vi "Agilent 546XX Series Acq Wfm Edge Triggered Oscilloscope Tapped.vi"(0 "VISA Resource Name":refnum<visa-resource-name> caption="VISA session", 1 "Vertical Coupling (DC)":i32(slide)=1, 2 "acquisition start time (0.0 sec)":dbl caption="Acquisition Start Time (0.0 sec)" format="%^.2e", 3 "probe attenuation (1.0)":dbl=1.0 caption="Probe Attenuation (1x)" format="%.2f", 5 "Channel Name (\"Channel 1\")":string(combo)="CHAN1", 7 "vertical range (40.0 V)":dbl=2.0 caption="Vertical Range (2.0 V)" format="%^.2e", 9 "time per record (1.00E-3 sec)":dbl=0.02 caption="Time Per Record (20.0E-3 sec)" format="%^.2e", 12 "trigger level (0.0 volts)":dbl caption="Trigger Level (0.0 volts)" format="%^.2e", 13 "minimum record length (2000)":i32=1000 caption="Min Record Length (1000 samples)", 14 "vertical offset (0.0 V)":dbl caption="Vertical Offset (0.0 V)" format="%^.2e") -> (6 "Waveform Graph":T1(graph))   [LabVIEW 2014]
doc: "DESCRIPTION:\nThis VI shows how to configure the ag546xx for a single-channel waveform acquisition. It uses edge triggering to trigger the acquisition. \n\nINSTRUCTIONS:\n1. Pass a valid instrument VISA session into this VI.\n2. Enter a vertical range and coupling for the specified channel.\n3. Enter the probe attenuation for the probe attached to the specified channel input.\n4. Enter the acquisition start time and desired time per record.\n5. Enter the trigger level for the edge trigger.\n6. Run the VI.\n7. The acquired waveform will be displayed in the graph.\n\nNOTES:\nNotice the order of the ag546xx component VIs in the block diagram. The first VI in this sequence accepts a valid instrument VISA session which provides a dup VISA session to the instrument driver. The instrument session is generated by the ag546xx Initialize.vi. The last VI in the sequence passes the VISA session out. \n\nThis VI sets the following controls on the block diagram:\n 60MHz Max Input Frequency.\n 1.0M Ohm Input Impedance.\n 200 ns Trigger Holdoff\n Edge trigger is DC coupled with a positive slope.\nTo change these values, modify the associated block diagram constants."
uses:
  <instrlib>/Agilent 546XX Series/Agilent 546XX Series.lvlib
panel:
  in  "Serial Configuration":cluster{"Baud Rate":u32, "Flow Control":u16}={"Baud Rate"=0, "Flow Control"=4} {"Flow Control" items=["None", "XON/XOFF", "RTS/CTS", "XON/XOFF & RTS/CTS", "DTR/DSR", "XON/XOFF & DTR/DSR"]; "Baud Rate" items=["9600", "19200", "38400", "57600"]}
  # "© 2003, National Instruments, Corporation.  All Rights Reserved."
  # "For instructions,\nselect Show Context Help\nfrom the Help menu."
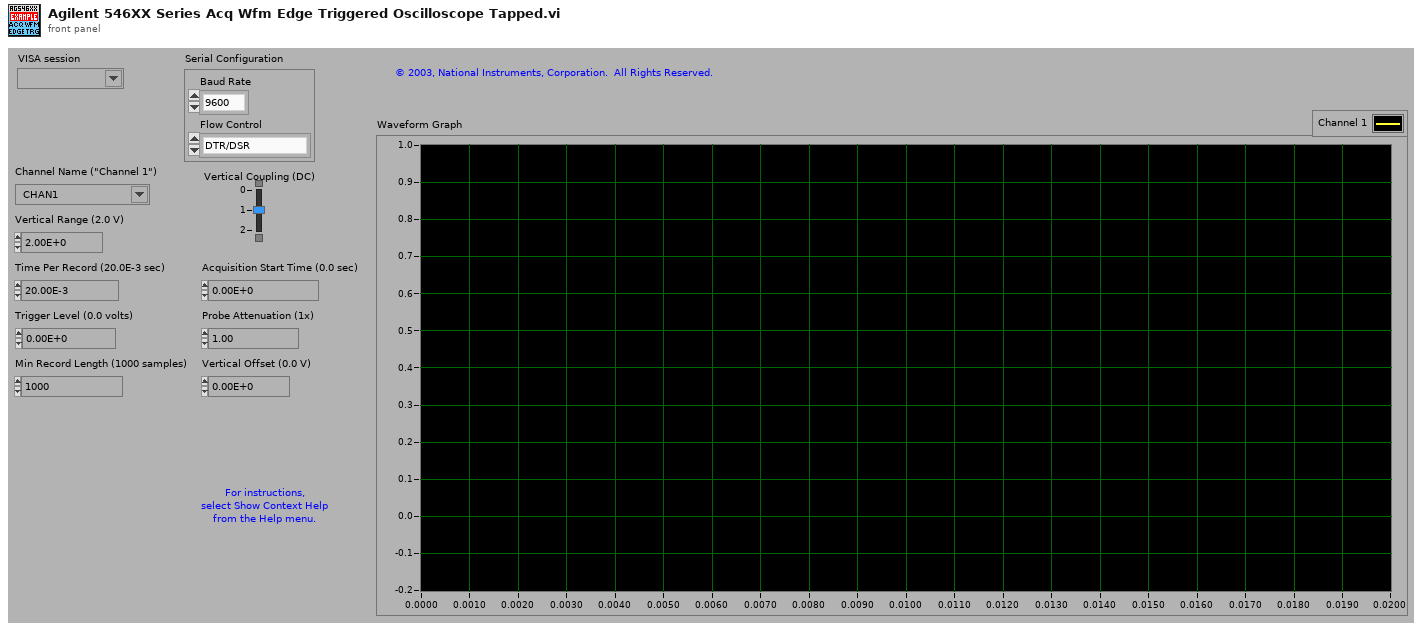
[diagram p1: front panel]
types:
  T1 = cluster{"Initial X":dbl, "X Increment":dbl, "Waveform Array":dbl[]}
  T2 = cluster{"initial x":dbl, "x increment":dbl, " waveform array  ":dbl[]}
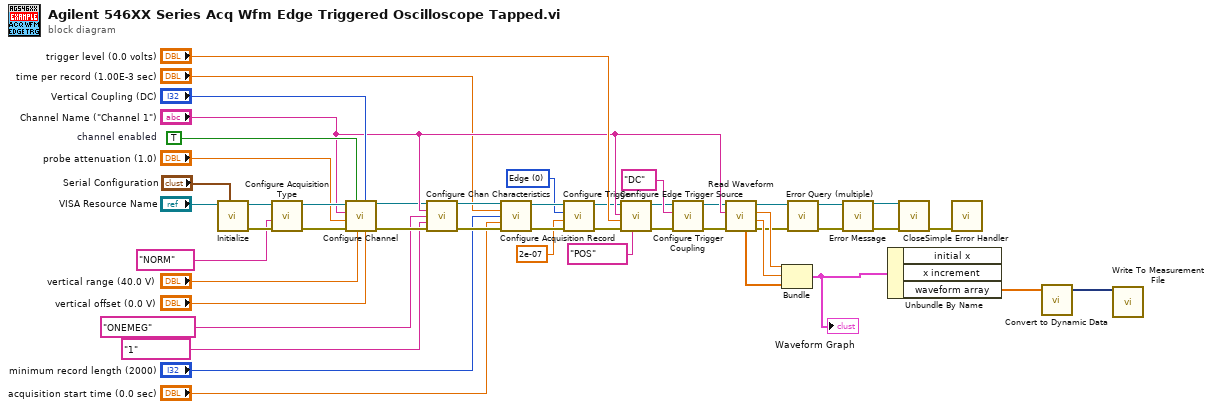
[diagram p0: block diagram]
diagram:
  w22 = 0 items=["Edge", "Glitch", "TV", "AC Line", "Pattern", "Duration", "IIC", "Sequence"] ("Trigger Type (Edge)")
  w39 = TRUE  # channel enabled
  n1 = call <instrlib>:"Initialize.vi"("Serial Configuration"="Serial Configuration", "VISA Resource Name"="VISA Resource Name") -> ("error out"=w48:errorcluster, "VISA Resource Name Out"=w12:refnum<visa-resource-name>)  [unwired: 8 in]
  n2 = call <instrlib>:"Configure Acquisition Type.vi"("error in (no error)"=w48, "Acquisition Type (Sample)"="NORM", "VISA Resource Name"=w12) -> ("error out"=w47:errorcluster, "VISA Resource Name Out"=w45:refnum<visa-resource-name>)  [unwired: 7 in]
  n3 = call <instrlib>:"Configure Channel.vi"("Vertical Offset (0.0 V)"="vertical offset (0.0 V)", "Vertical Coupling (DC)"="Vertical Coupling (DC)", "Vertical Range (40 V)"="vertical range (40.0 V)", "Channel Enabled (True)"=w39, "error in (no error)"=w47, "Probe Attenuation (1x)"="probe attenuation (1.0)", "Channel Name (\"Channel 1\")"="Channel Name (\"Channel 1\")", "VISA Resource Name"=w45) -> ("error out"=w46:errorcluster, "VISA Resource Name Out"=w26:refnum<visa-resource-name>)  [unwired: 2 in]
  n4 = call <instrlib>:"Configure Chan Characteristics.vi"("VISA Resource Name"=w26, "Channel Name (\"Channel 1\")"="Channel Name (\"Channel 1\")", "Input Impedance (1.0 mega ohm)"="ONEMEG", "Max Input Frequency (20.0E+6 Hz)"="1", "error in (no error)"=w46) -> ("VISA Resource Name Out"=w34:refnum<visa-resource-name>, "error out"=w32:errorcluster)  [unwired: 9 in]
  n5 = call <instrlib>:"Configure Acquisition Record.vi"("VISA Resource Name"=w34, "Time Per Record (1.0e-3 s)"="time per record (1.00E-3 sec)", "Minimum Record Length (2000)"="minimum record length (2000)", "Acquisition Start Time (0.0 s)"="acquisition start time (0.0 sec)", "error in (no error)"=w32) -> ("VISA Resource Name Out"=w28:refnum<visa-resource-name>, "error out"=w29:errorcluster)  [unwired: 9 in]
  n6 = call <instrlib>:"Configure Trigger.vi"("error in (no error)"=w29, "trigger holdoff (60.0E-9 s)"=2e-07, "Trigger Type (Edge)"=w22, "VISA Resource Name"=w28) -> ("error out"=w18:errorcluster, "VISA Resource Name Out"=w19:refnum<visa-resource-name>)  [unwired: 6 in]
  n7 = call <instrlib>:"Configure Edge Trigger Source.vi"("Trigger Slope (Positive)"="POS", "error in (no error)"=w18, "Trigger Level (0.0 V)"="trigger level (0.0 volts)", "Trigger Source (Channel 1)"="Channel Name (\"Channel 1\")", "VISA Resource Name"=w19) -> ("error out"=w16:errorcluster, "VISA Resource Name Out"=w17:refnum<visa-resource-name>)  [unwired: 5 in]
  n8 = call <instrlib>:"Configure Trigger Coupling.vi"("error in (no error)"=w16, "Trigger Coupling (DC)"="DC", "VISA Resource Name"=w17) -> ("error out"=w14:errorcluster, "VISA Resource Name Out"=w15:refnum<visa-resource-name>)  [unwired: 7 in]
  n9 = call <instrlib>:"Read Waveform.vi"("error in (no error)"=w14, "Channel Name (\"Channel 1\")"="Channel Name (\"Channel 1\")", "VISA Resource Name"=w15) -> ("error out"=w10:errorcluster, "x increment"=w36:dbl, "initial x"=w37:dbl, "VISA Resource Name Out"=w11:refnum<visa-resource-name>, "waveform array"=w38:dbl[])  [unwired: 3 in, 1 out]
  n10 = Bundle("initial x"=w37, "x increment"=w36, "waveform array"=w38) -> (w3:T2)  [unwired: 1 in]
  "Waveform Graph" <- w3
  n11 = call <instrlib>:"Error Query (multiple).vi"("error in (no error)"=w10, "VISA Resource Name"=w11) -> ("error out"=w8:errorcluster, "VISA Resource Name Out"=w9:refnum<visa-resource-name>)  [unwired: 6 in, 2 out]
  n12 = call <instrlib>:"Error Message.vi"("VISA Resource Name"=w9, "error in (no error)"=w8) -> ("VISA Resource Name Out"=w7:refnum<visa-resource-name>, "error out"=w6:errorcluster)  [unwired: 9 in, 3 out]
  n13 = Unbundle By Name(w3) -> ("waveform array"=w1:dbl[])  [unwired: 2 out]
  n14 = call <instrlib>:"Close.vi"("error in (no error)"=w6, "VISA Resource Name"=w7) -> ("error out"=w5:errorcluster)  [unwired: 9 in]
  n15 = call <vilib>:"Simple Error Handler.vi"("error in (no error)"=w5) -> ()  [unwired: 4 in, 5 out]
  n16 = call "Convert to Dynamic Data"("Array"=w1) -> ("Dynamic Data Type"=w2:dynamicdata)  [unwired: 3 in]
  n17 = call "Write To Measurement File"("Signals"=w2) -> ()  [unwired: 16 in, 3 out]
